vi "Candidate Selection Testing.vi"() -> ()   [LabVIEW 2016]
uses:
  <vilib>/vision/NI_Vision_Development_Module.lvlib
panel:
  out "And Image":T1(plugin-control)
  out "Sub Over Dilated":T1(plugin-control)
  out "Dilated Image":T1(plugin-control)
  out "Input Image":T1(plugin-control)
  out "Conv with 3 x 3":T1(plugin-control)
  out "Conv with 9 x 9":T1(plugin-control)
  out "Subtracted Image":T1(plugin-control)
  out "Threshold Image":T1(plugin-control)
  in  "Image to Read":path=path "Z:/Edward/Drift Correction/Test Data/Egg Chamber Test Data/Stack02/Color02/Color02_00001.tif"
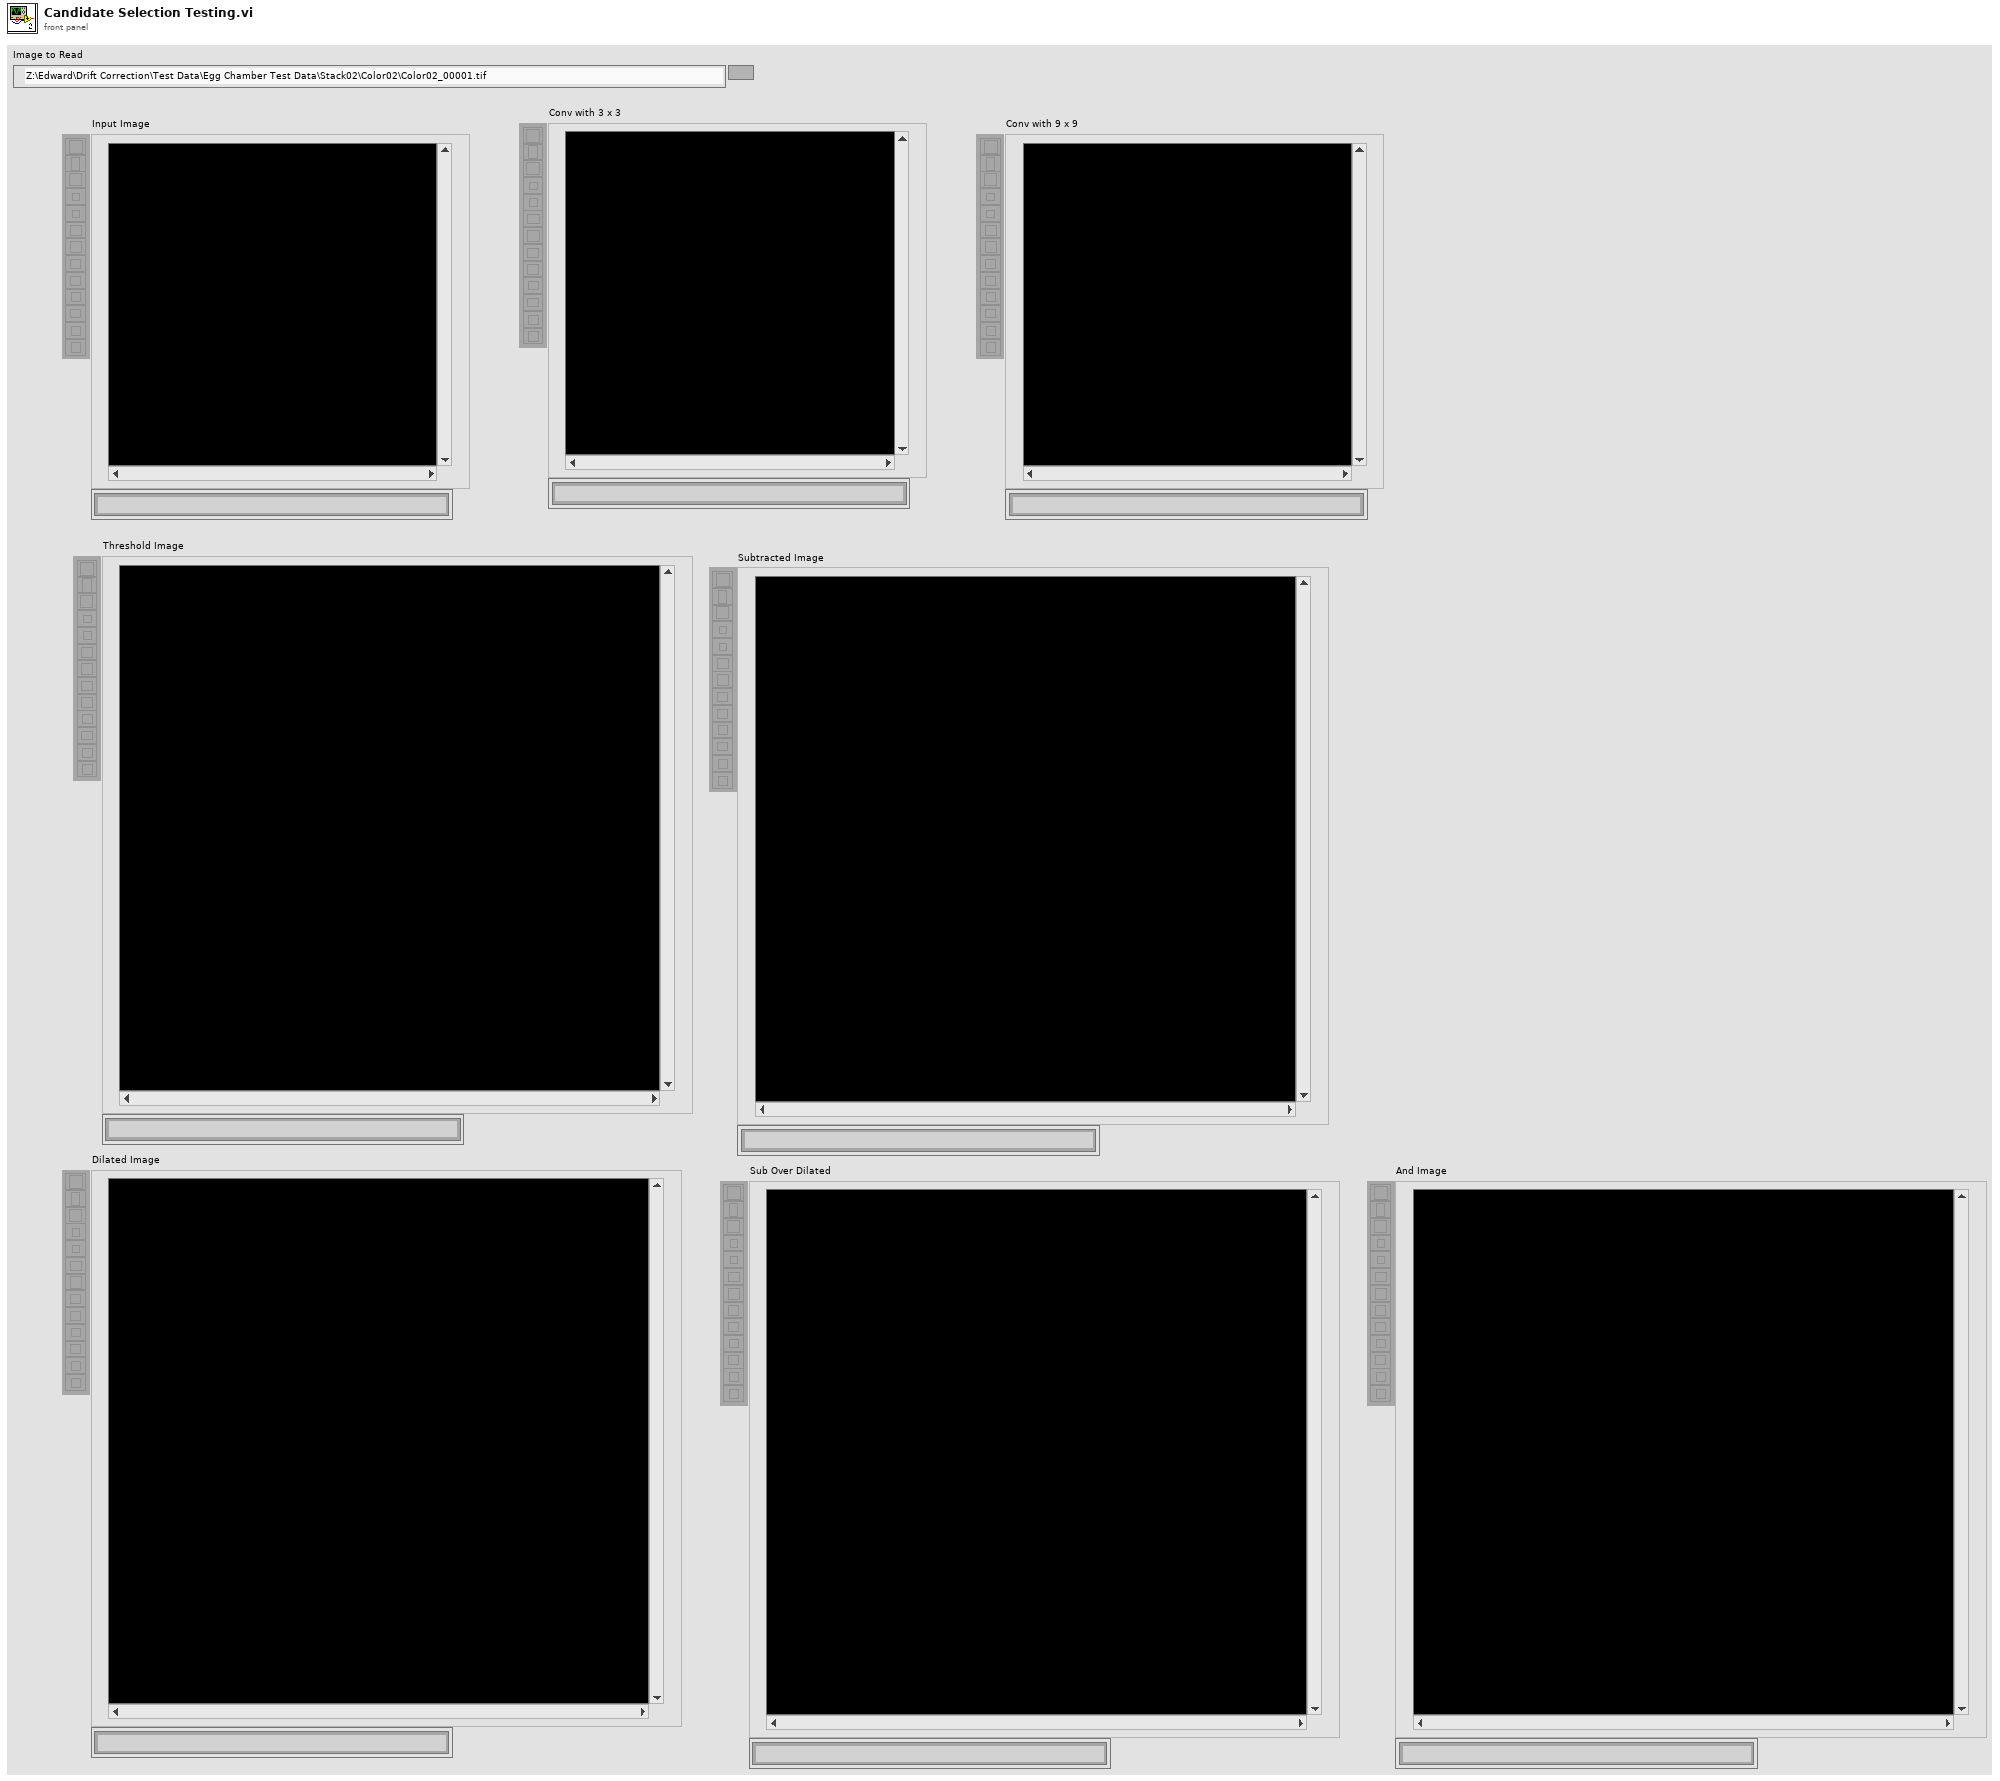
[diagram p1: front panel]
types:
  T1 = typedef "IMAQ Image.ctl" = refnum<image>
  T2 = typedef "Image Type" = u32
  T3 = enum32{"Average", "Min", "Max", "Clear  if < ", "Clear  if < or =", "Clear  if =", "Clear  if > or =", "Clear  if >"}
  T4 = enum32{"AutoM", "Close", "Dilate", "Erode", "Gradient", "Gradient in", "Gradient out", "HitMiss", "Open", "PClose", "POpen", "Thick", "Thin"}
  T5 = cluster{"histogram":u32[], "Minimal Value":sgl, "Maximal Value":sgl, "Starting Value":sgl, "Interval Width":sgl, "Mean Value":sgl, "Standard  Variation":sgl, "Area (pixels)":i32}
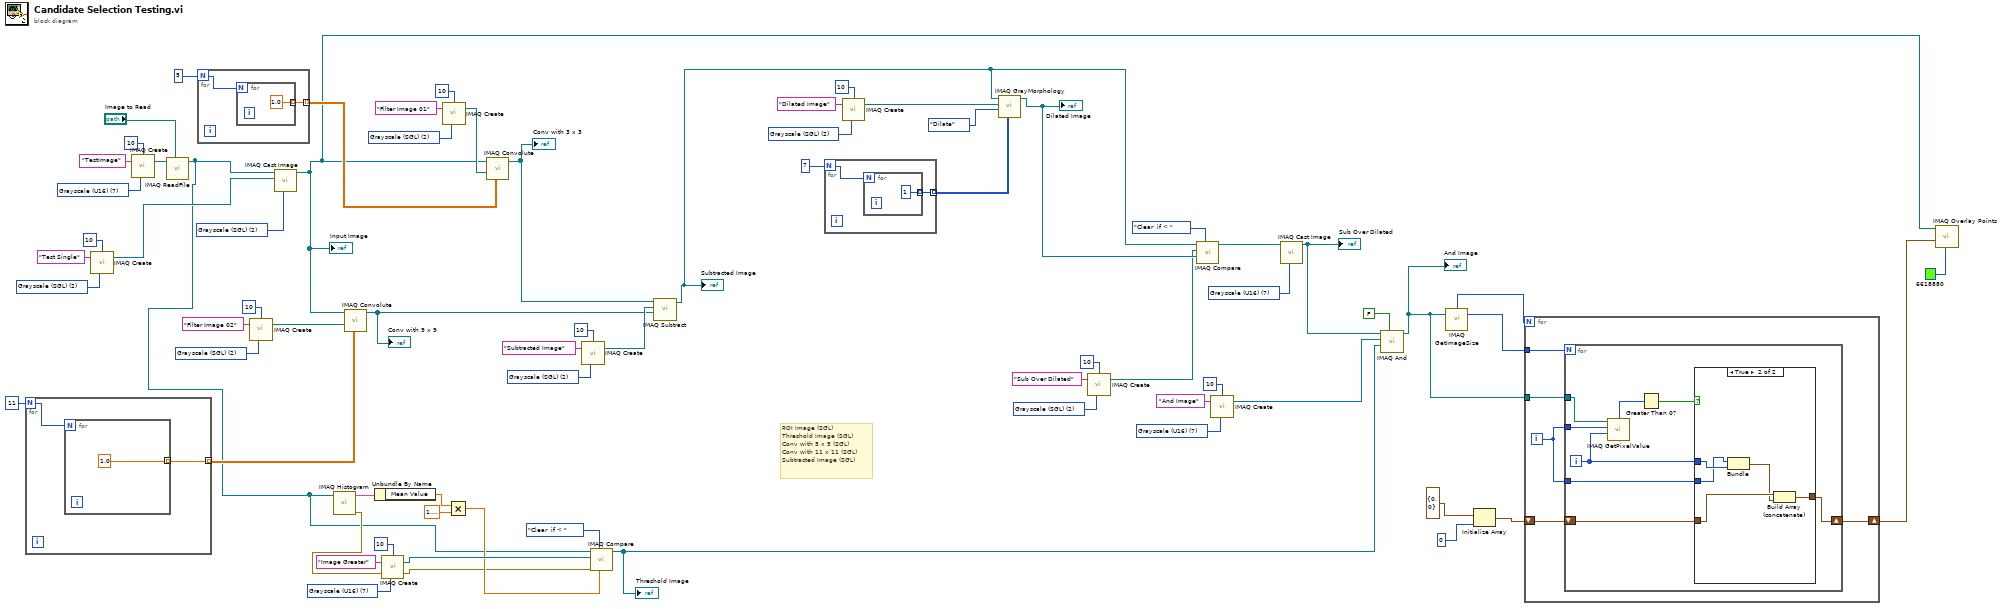
[diagram p0: block diagram]
diagram:
  w11 = T2 7 items=["Grayscale (U8)", "Grayscale (I16)", "Grayscale (SGL)", "Complex (CSG)", "RGB (U32)", "HSL (U32)", "RGB (U64)", "Grayscale (U16)"] ("Image Type")
  w19 = T2 7 items=["Grayscale (U8)", "Grayscale (I16)", "Grayscale (SGL)", "Complex (CSG)", "RGB (U32)", "HSL (U32)", "RGB (U64)", "Grayscale (U16)"] ("Image Type")
  w23 = T2 2 items=["Grayscale (U8)", "Grayscale (I16)", "Grayscale (SGL)", "Complex (CSG)", "RGB (U32)", "HSL (U32)", "RGB (U64)", "Grayscale (U16)"] ("Image Type")
  w32 = T2 2 items=["Grayscale (U8)", "Grayscale (I16)", "Grayscale (SGL)", "Complex (CSG)", "RGB (U32)", "HSL (U32)", "RGB (U64)", "Grayscale (U16)"] ("Image Type")
  w44 = T2 7 items=["Grayscale (U8)", "Grayscale (I16)", "Grayscale (SGL)", "Complex (CSG)", "RGB (U32)", "HSL (U32)", "RGB (U64)", "Grayscale (U16)"] ("Image Type")
  w52 = T2 2 items=["Grayscale (U8)", "Grayscale (I16)", "Grayscale (SGL)", "Complex (CSG)", "RGB (U32)", "HSL (U32)", "RGB (U64)", "Grayscale (U16)"] ("Image Type")
  w55 = T2 2 items=["Grayscale (U8)", "Grayscale (I16)", "Grayscale (SGL)", "Complex (CSG)", "RGB (U32)", "HSL (U32)", "RGB (U64)", "Grayscale (U16)"] ("Image Type")
  w57 = T2 2 items=["Grayscale (U8)", "Grayscale (I16)", "Grayscale (SGL)", "Complex (CSG)", "RGB (U32)", "HSL (U32)", "RGB (U64)", "Grayscale (U16)"] ("Image Type")
  w64 = T2 2 items=["Grayscale (U8)", "Grayscale (I16)", "Grayscale (SGL)", "Complex (CSG)", "RGB (U32)", "HSL (U32)", "RGB (U64)", "Grayscale (U16)"] ("Image Type")
  w65 = T2 2 items=["Grayscale (U8)", "Grayscale (I16)", "Grayscale (SGL)", "Complex (CSG)", "RGB (U32)", "HSL (U32)", "RGB (U64)", "Grayscale (U16)"] ("Image Type")
  w71 = T2 7 items=["Grayscale (U8)", "Grayscale (I16)", "Grayscale (SGL)", "Complex (CSG)", "RGB (U32)", "HSL (U32)", "RGB (U64)", "Grayscale (U16)"] ("Image Type")
  # "ROI Image (SGL)\nThreshold Image (SGL)\nConv with 5 x 5 (SGL)\nConv with 11 x 11 (SGL)\nSubtracted Image (SGL)"
  n1 = for {
    N: 11 -> [w73]
    tunnel: [w74] -> w49 mode=indexing
    n2 = for {
      N: w73 -> [_]
      tunnel: [sgl 1.0] -> w74 mode=indexing
    }
  }
  n3 = call "IMAQ Create"("Border Size"=10, "Image Name"="Test Single", "Image Type"=w52) -> ("New Image"=w51:T1)  [unwired: 2 in, 1 out]
  n4 = call "IMAQ Create"("Border Size"=10, "Image Name"="TestImage", "Image Type"=w71) -> ("New Image"=w72:T1)  [unwired: 2 in, 1 out]
  n5 = call "IMAQ ReadFile"("File Path"="Image to Read", "Image"=w72) -> ("Image Out"=w13:T1)  [unwired: 5 in, 4 out]
  n6 = for {
    N: 5 -> [w76]
    tunnel: [w77] -> w47 mode=indexing
    n7 = for {
      N: w76 -> [_]
      tunnel: [sgl 1.0] -> w77 mode=indexing
    }
  }
  n8 = call "IMAQ Create"("Border Size"=10, "Image Name"="Filter Image 02", "Image Type"=w64) -> ("New Image"=w60:T1)  [unwired: 2 in, 1 out]
  n9 = call "IMAQ Cast Image"("Image Type"=w55, "Image Dst"=w51, "Image Src"=w13) -> ("Image Dst Out"=w3:T1)  [unwired: 7 in, 1 out]
  "Input Image" <- w3
  n10 = call "IMAQ Histogram"("Image"=w13) -> ("error out"=w35:errorcluster, "Histogram Report"=w41:T5)  [unwired: 9 in]
  n11 = call "IMAQ Convolute"("Kernel"=w49, "Image Dst"=w60, "Image Src"=w3) -> ("Image Dst Out"=w37:T1)  [unwired: 7 in, 1 out]
  "Conv with 9 x 9" <- w37
  n12 = Unbundle By Name(w41) -> ("Mean Value"=w40:sgl)
  n13 = call "IMAQ Create"("Border Size"=10, "Image Name"="Image Greater", "Image Type"=w44, "error in (no error)"=w35) -> ("New Image"=w42:T1, "error out"=w34:errorcluster)  [unwired: 1 in]
  n14 = call "IMAQ Create"("Border Size"=10, "Image Name"="Filter Image 01", "Image Type"=w65) -> ("New Image"=w61:T1)  [unwired: 2 in, 1 out]
  n15 = Multiply(x=w40, y=sgl 1.2) -> (x*y=w38:sgl)
  n16 = call "IMAQ Convolute"("Kernel"=w47, "Image Dst"=w61, "Image Src"=w3) -> ("Image Dst Out"=w36:T1)  [unwired: 7 in, 1 out]
  "Conv with 3 x 3" <- w36
  n17 = call "IMAQ Create"("Border Size"=10, "Image Name"="Subtracted Image", "Image Type"=w57) -> ("New Image"=w56:T1)  [unwired: 2 in, 1 out]
  n18 = call "IMAQ Compare"("Constant"=w38, "Operator"=T3."Clear  if < ", "error in (no error)"=w34, "Image Dst"=w42, "Image Src A"=w13) -> ("Image Dst Out"=w14:T1)  [unwired: 5 in, 1 out]
  "Threshold Image" <- w14
  n19 = call "IMAQ Subtract"("Image Src A"=w36, "Image Dst"=w56, "Image Src B"=w37) -> ("Image Dst Out"=w15:T1)  [unwired: 4 in, 1 out]
  "Subtracted Image" <- w15
  n20 = for {
    N: 7 -> [w79]
    tunnel: [w80] -> w27 mode=indexing
    n21 = for {
      N: w79 -> [_]
      tunnel: [1] -> w80 mode=indexing
    }
  }
  n22 = call "IMAQ Create"("Border Size"=10, "Image Name"="Dilated Image", "Image Type"=w32) -> ("New Image"=w31:T1)  [unwired: 2 in, 1 out]
  n23 = call "IMAQ GrayMorphology"("Structuring Element"=w27, "Operation"=T4."Dilate", "Image Dst"=w31, "Image Src"=w15) -> ("Image Dst Out"=w25:T1)  [unwired: 6 in, 1 out]
  "Dilated Image" <- w25
  n24 = call "IMAQ Create"("Border Size"=10, "Image Name"="Sub Over Dilated", "Image Type"=w23) -> ("New Image"=w21:T1)  [unwired: 2 in, 1 out]
  n25 = call "IMAQ Compare"("Operator"=T3."Clear  if < ", "Image Src B"=w25, "Image Dst"=w21, "Image Src A"=w15) -> ("Image Dst Out"=w12:T1)  [unwired: 6 in, 1 out]
  n26 = call "IMAQ Create"("Border Size"=10, "Image Name"="And Image", "Image Type"=w19) -> ("New Image"=w17:T1)  [unwired: 2 in, 1 out]
  n27 = call "IMAQ Cast Image"("Image Type"=w11, "Image Src"=w12) -> ("Image Dst Out"=w10:T1)  [unwired: 8 in, 1 out]
  "Sub Over Dilated" <- w10
  n28 = call "IMAQ And"("And/Nand (And)"=FALSE, "Image Src B"=w14, "Image Dst"=w17, "Image Src A"=w10) -> ("Image Dst Out"=w5:T1)  [unwired: 6 in, 1 out]
  "And Image" <- w5
  n29 = call "IMAQ GetImageSize"("Image"=w5) -> ("Y Resolution"=w8:i32, "X Resolution"=w9:i32)  [unwired: 3 in, 1 out]
  n30 = Initialize Array(cluster{"X":i32, "Y":i32} {"X"=0, "Y"=0} ("Point"), 0 ("element")) -> (w6:cluster{"X":i32, "Y":i32}[])
  n31 = for {
    N: w9 -> [_]
    tunnel: w8 -> [w86]
    shift-right: [w83] -> w1
    shift-left: w6 -> [w84]
    tunnel: w5 -> [w82]
    i -> [w85]
    n32 = for {
      N: w86 -> [_]
      tunnel: w85 -> [w94]
      tunnel: w85 -> [w91]
      tunnel: w82 -> [w88]
      shift-right: [w89] -> w83
      shift-left: w84 -> [w90]
      i -> [w92]
      n33 = call "IMAQ GetPixelValue"("Image"=w88, "X Coordinate"=w94, "Y Coordinate"=w92) -> ("Pixel Value (U16)"=w87:u16)  [unwired: 3 in, 4 out]
      n34 = Greater Than 0?(x=w87) -> (x > 0?=w93:bool)
      n35 = case shown="True" w93 {
        tunnel: w92 -> [_ w97]
        tunnel: w91 -> [_ w96]
        tunnel: w90 -> [w95 w100]
        tunnel: [w95 w99] -> w89
        frame False {
        }
        frame True {
          n36 = Bundle(w96, w97) -> (w98:cluster{i32, i32})  [unwired: 1 in]
          n37 = Build Array (concatenate)(w100, w98) -> (w99:cluster{"X":i32, "Y":i32}[])
        }
      }
    }
  }
  n38 = call "IMAQ Overlay Points"("Color"=u32 6618880, "Array of Points"=w1, "Image"=w3) -> ()  [unwired: 7 in, 2 out]
